vi "ShutterControl.vi"() -> ()   [LabVIEW 2019]
uses:
  <vilib>/DAQmx/write.llb/DAQmx Write (Analog DBL 1Chan 1Samp).vi
  <vilib>/DAQmx/miscellaneous.llb/DAQmx Fill In Error Info.vi
  <vilib>/DAQmx/create/channels.llb/DAQmx Create Channel (AO-Voltage-Basic).vi
  <vilib>/Analysis/1siggen.llb/Ramp Pattern by Delta.vi
  Driver/Newport ESP301/Newport ESP301.lvlib
  <vilib>/Analysis/NI_AALBase.lvlib
panel:
  in  "Dwell_positions":string[][](table)=[["-500", "3000"], ["-100", "3000"], ["0", "5000"], ["100", "5000"], ["500", "5000"], ["750", "10000"], ["1000", "10000"], ["", ""]]
  in  "Enable2":bool caption="Enable?"
  in  "Wait time [ms]":u32=1000 caption="Values <50 \nwon't work"
  out "StepSize [mm]":dbl=0.14989622900000002
  in  "stop 2":bool
  in  "StepSize [fs]":i32=1000
  in  "Enable?":bool
  out "a":waveform(dbl)(graph)={"t0"=timestamp(3675940489.011235 s since 1904-01-01), "dt"=1.0, "Y"=[-33.8895]}
  out "Waveform Chart":dbl(graph)=5.25341140860948
  out "x*y":dbl=-876.4751437142558
  in  "physical channels":tag="Dev1/ao1"
  out "DAC error":errorcluster
  out "ESP error":errorcluster
  out "run?":bool
  in  "set_vel":bool
  in  "velocity [fs/s]":dbl=333.564095198152
  in  "vel_mm":dbl=0.005 caption="velocity [mm/s]"
  out "meas. velocity":dbl
  in  "stop":bool
  out "output voltage":dbl
  in  "start":bool
  in  "go2p1":bool
  out "position [mm]":dbl=-33.8895
  in  "p2 [mm]":dbl=-0.707153771
  in  "p1 [mm]":dbl=-1.006946229
  in  "interpolate output":bool
  in  "Delta2 [fs]":dbl=999.9999999999999
  in  "Delta1 [fs]":dbl=-999.9999999999999
  in  "Reference [mm]":dbl=-0.85705
  in  "Axis (1)":i32=3 min=1 max=3
  in  "Serial Link (RS232)":enum16{"RS232", "USB"}(ring)
  in  "VISA resource name":refnum<visa-resource-name>="COM8"
  in  "main_close":bool
  # "Interface panel"
  # "Velocity panel"
  # "Positions panel"
  # "Equally spaced steps panel"
  # "Controls panel"
  # "User-defined steps panel"
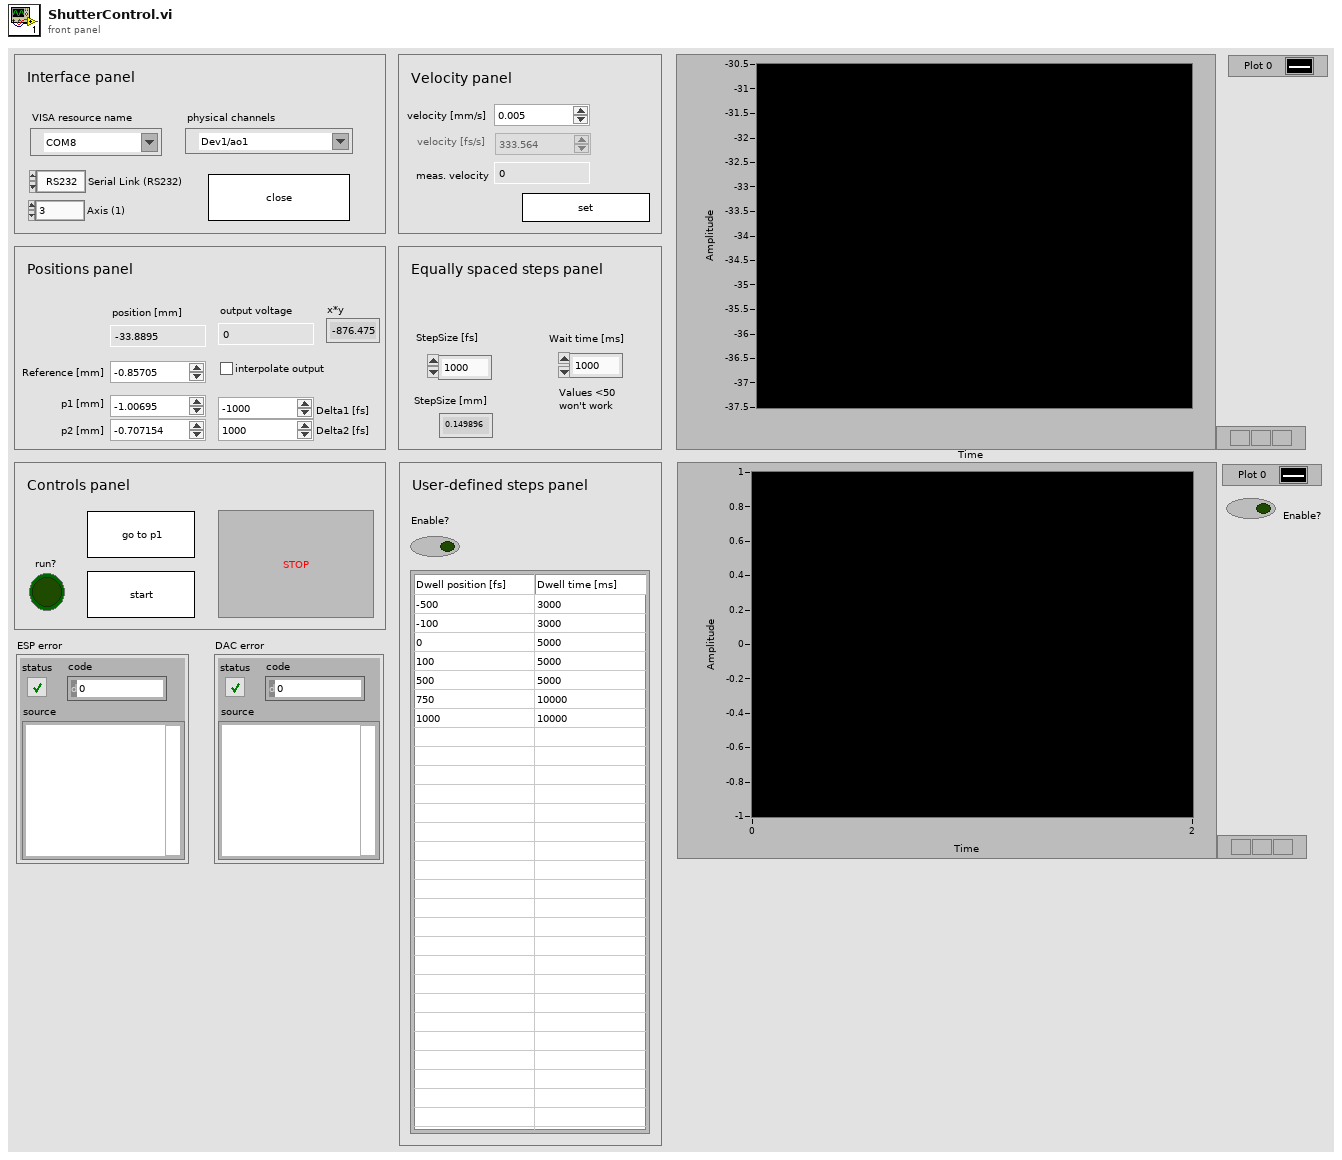
[diagram p1: front panel]
types:
  T1 = cluster{"dev1_data":refnum<queue>, "dev2_data":refnum<queue>}
  T2 = cluster{"dev1_cmd":refnum<queue>, "dev2_cmd":refnum<queue>}
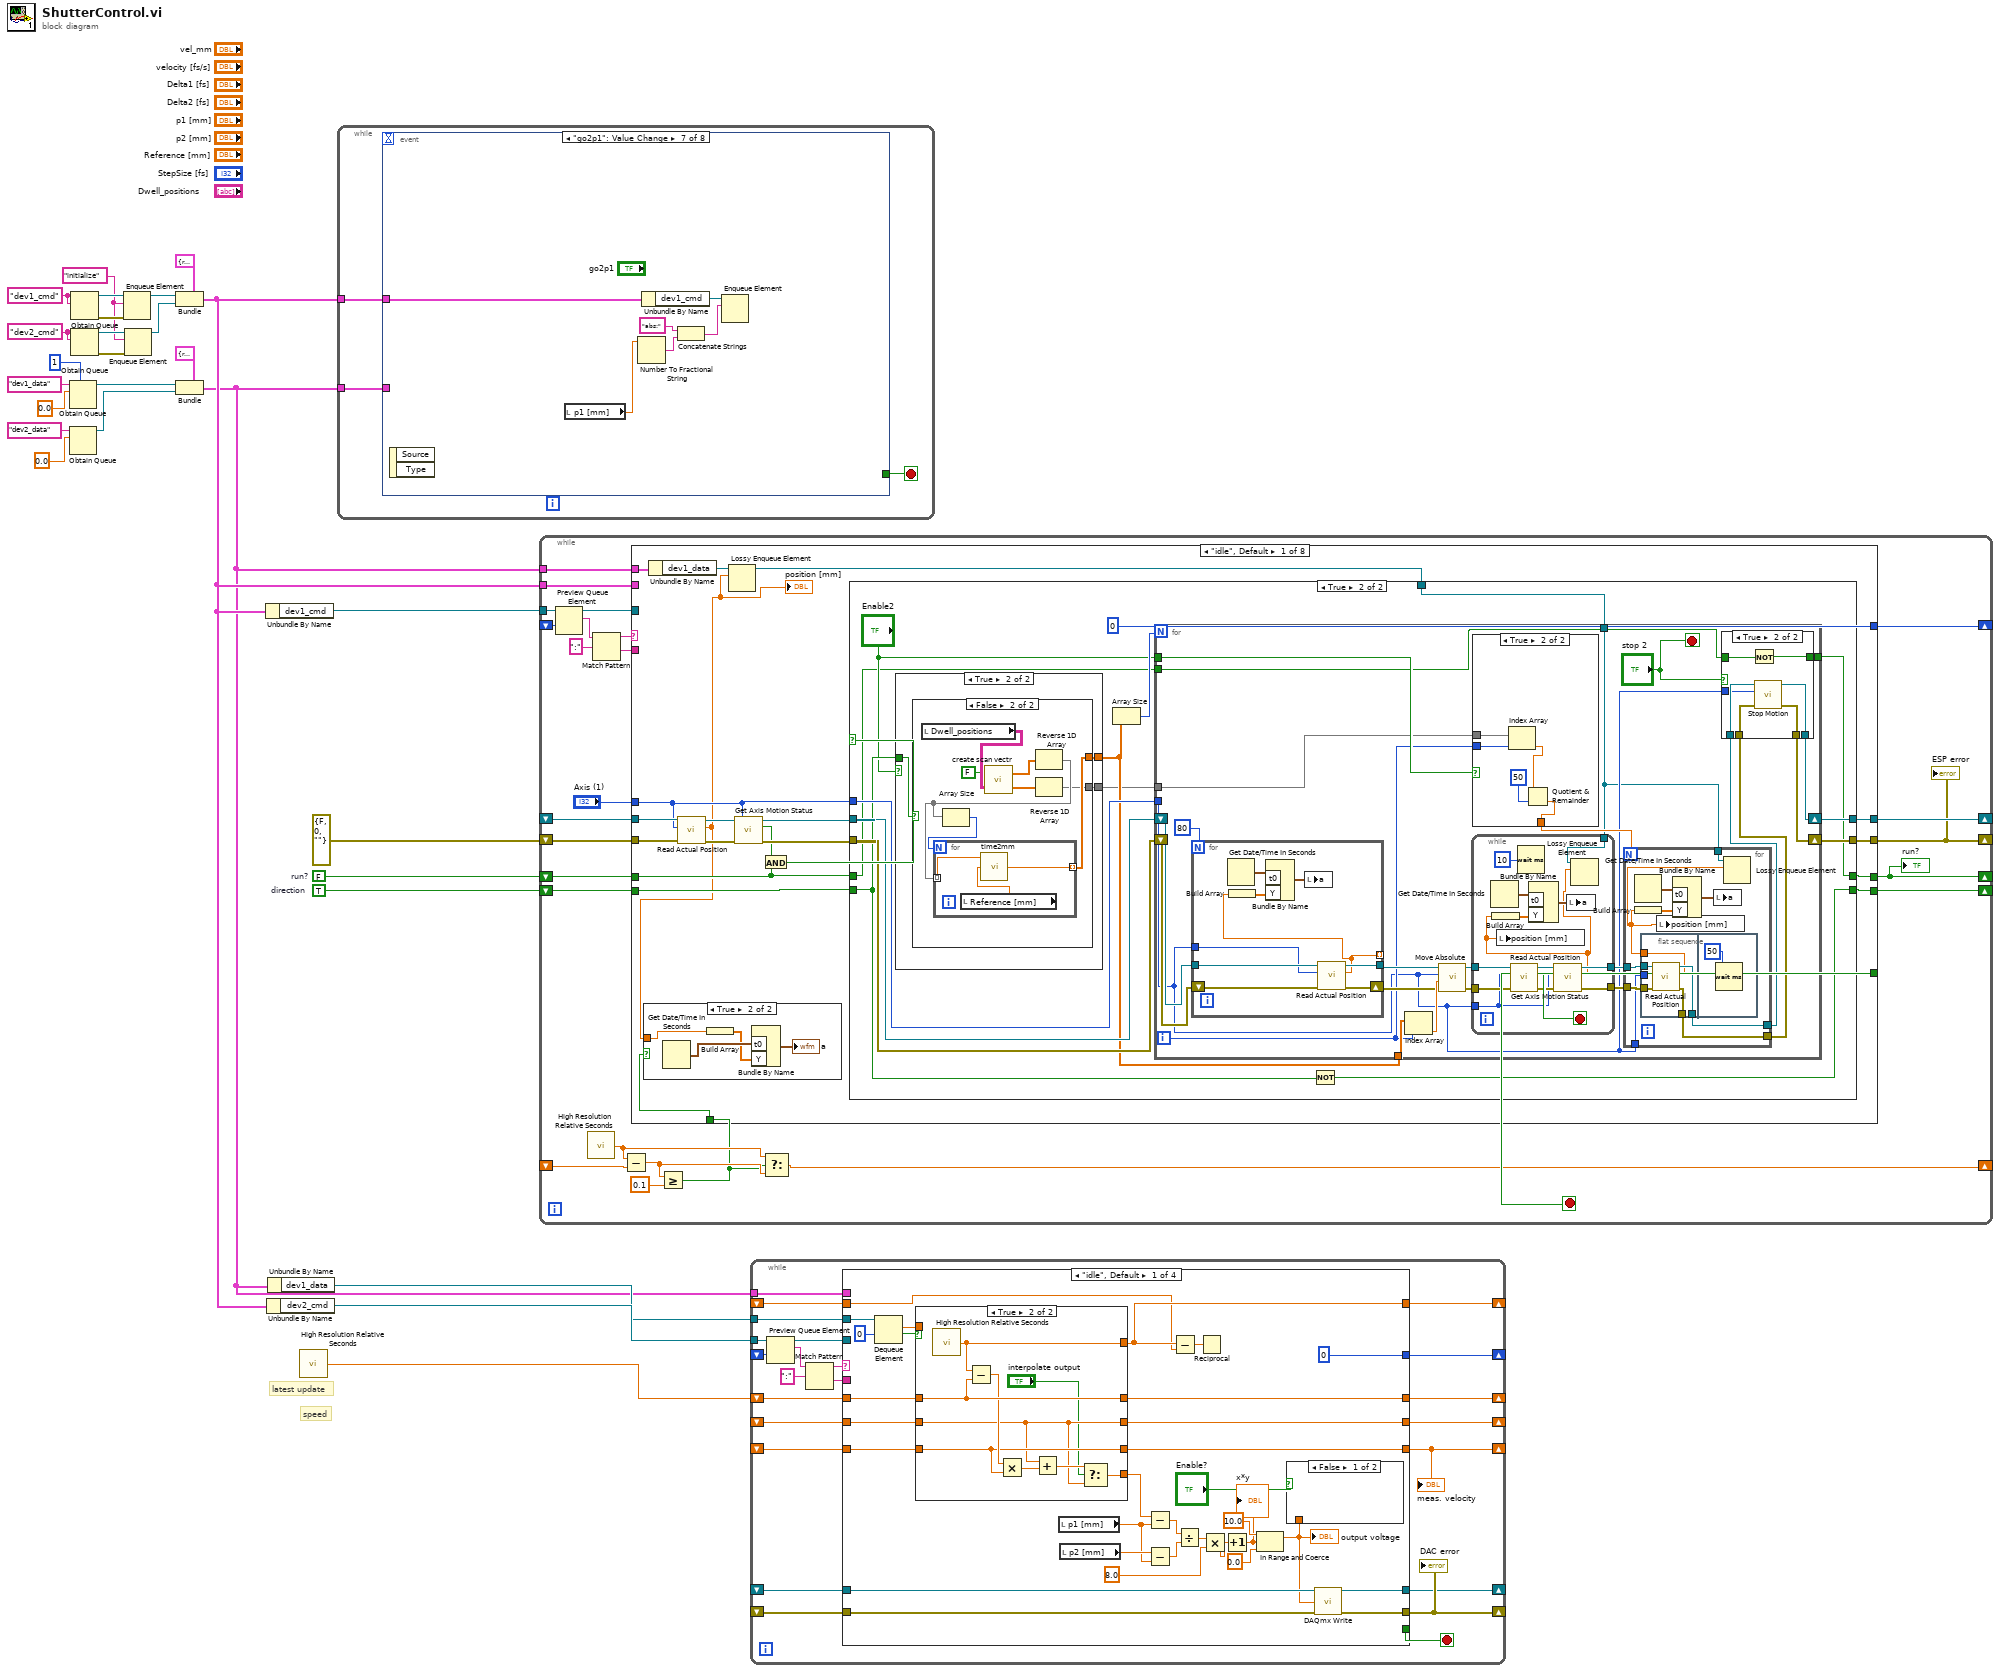
[diagram p0: block diagram]
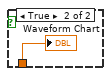
[diagram p2: hidden frame]
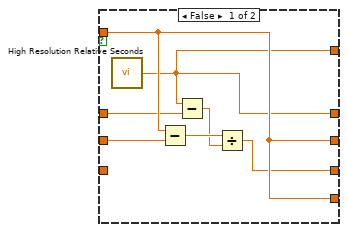
[diagram p3: hidden frame]
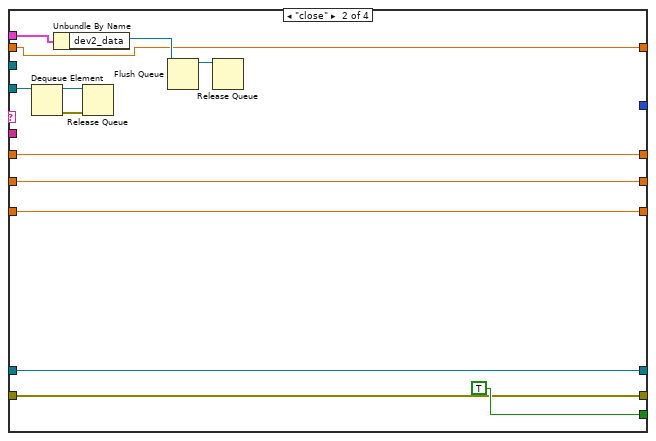
[diagram p4: hidden frame]
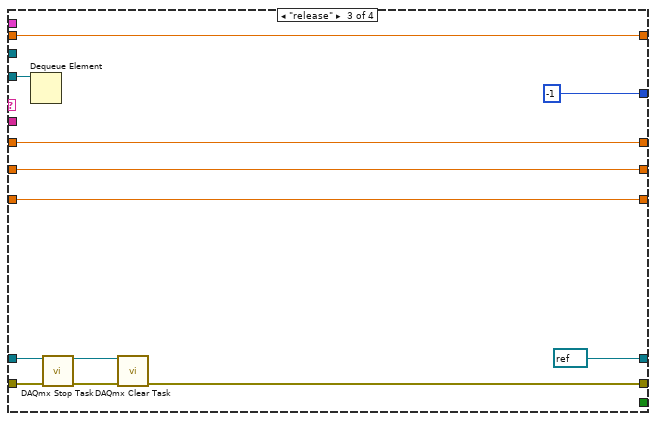
[diagram p5: hidden frame]
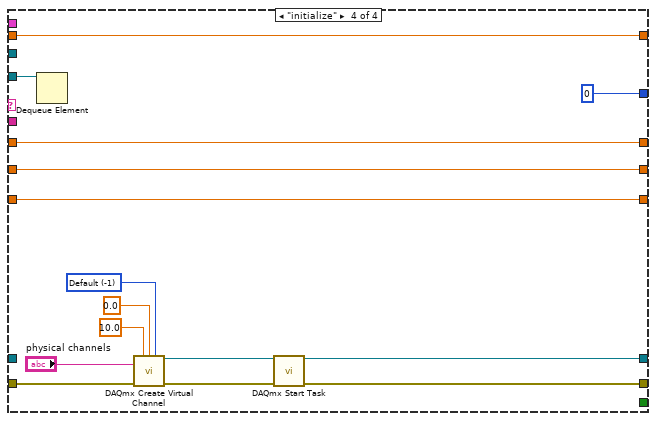
[diagram p6: hidden frame]
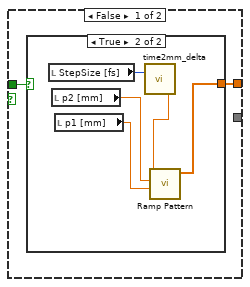
[diagram p9: hidden frame]
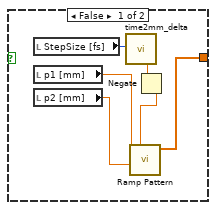
[diagram p10: hidden frame]
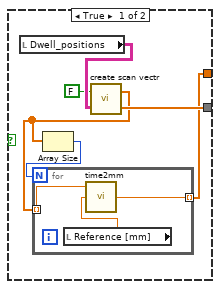
[diagram p11: hidden frame]
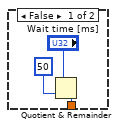
[diagram p13: hidden frame]
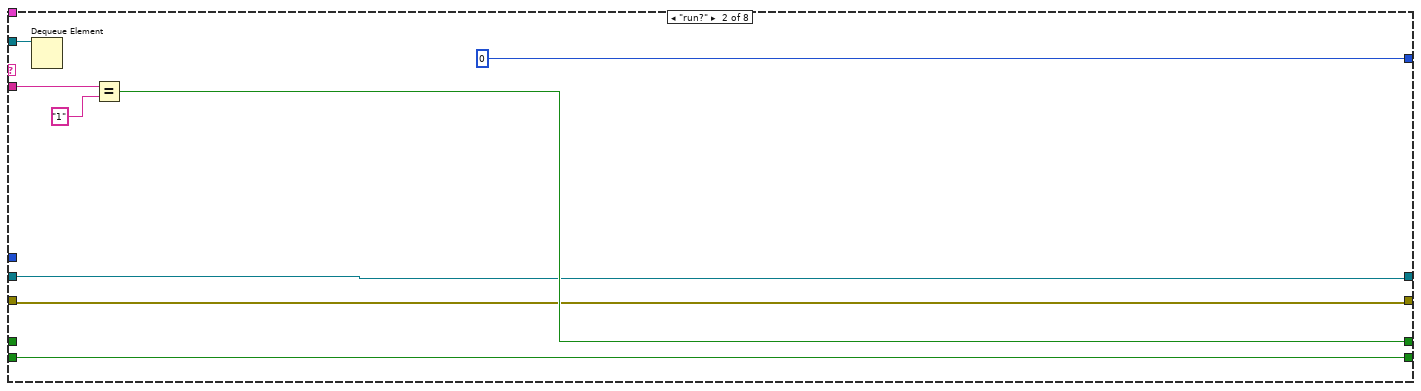
[diagram p14: hidden frame]
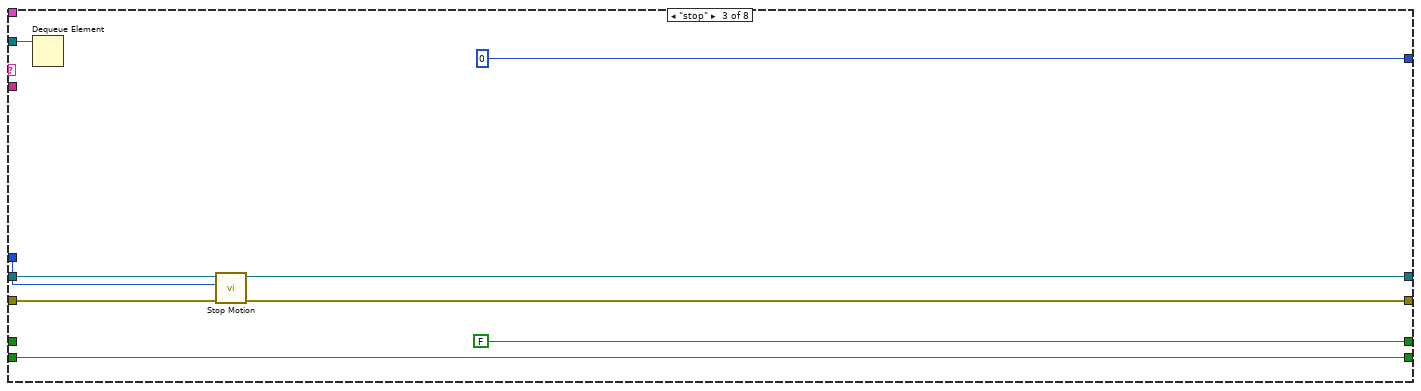
[diagram p15: hidden frame]
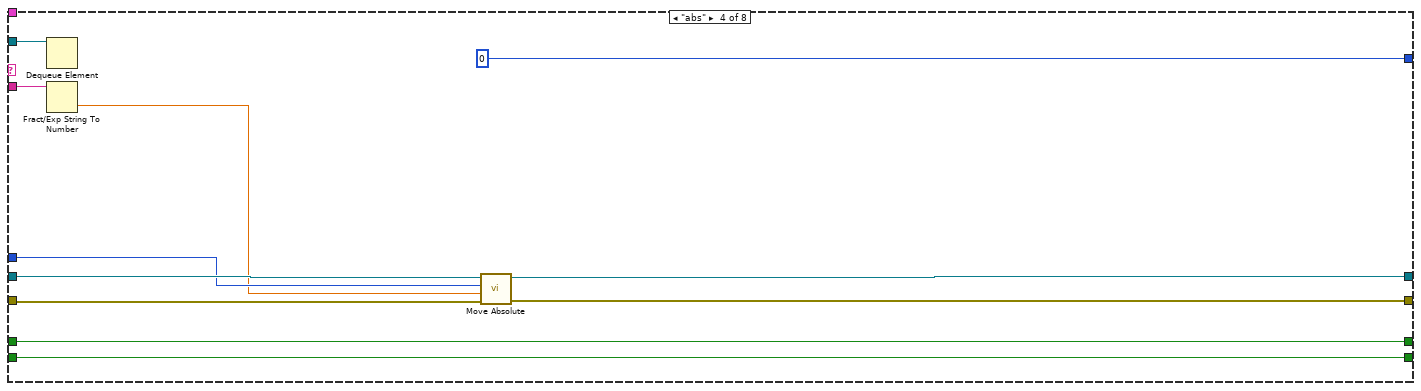
[diagram p16: hidden frame]
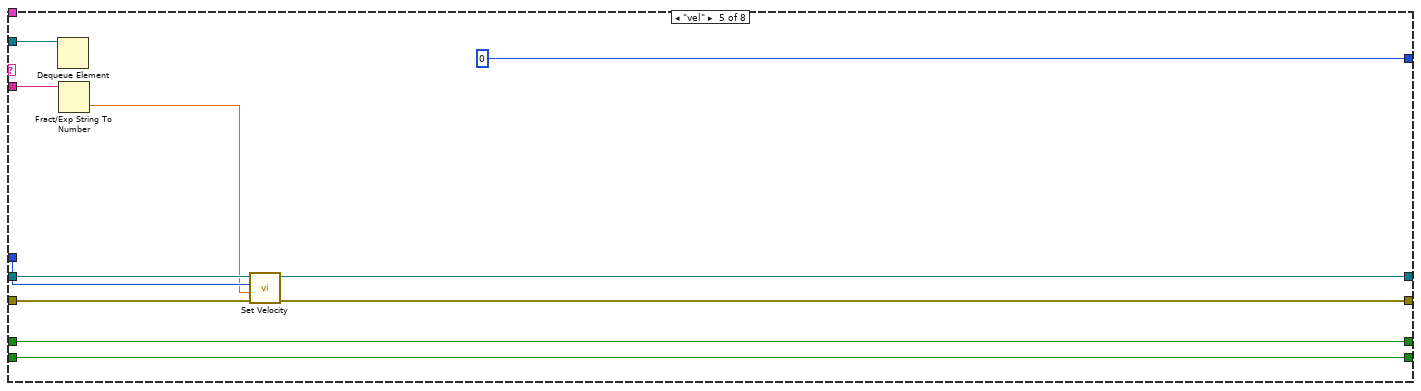
[diagram p17: hidden frame]
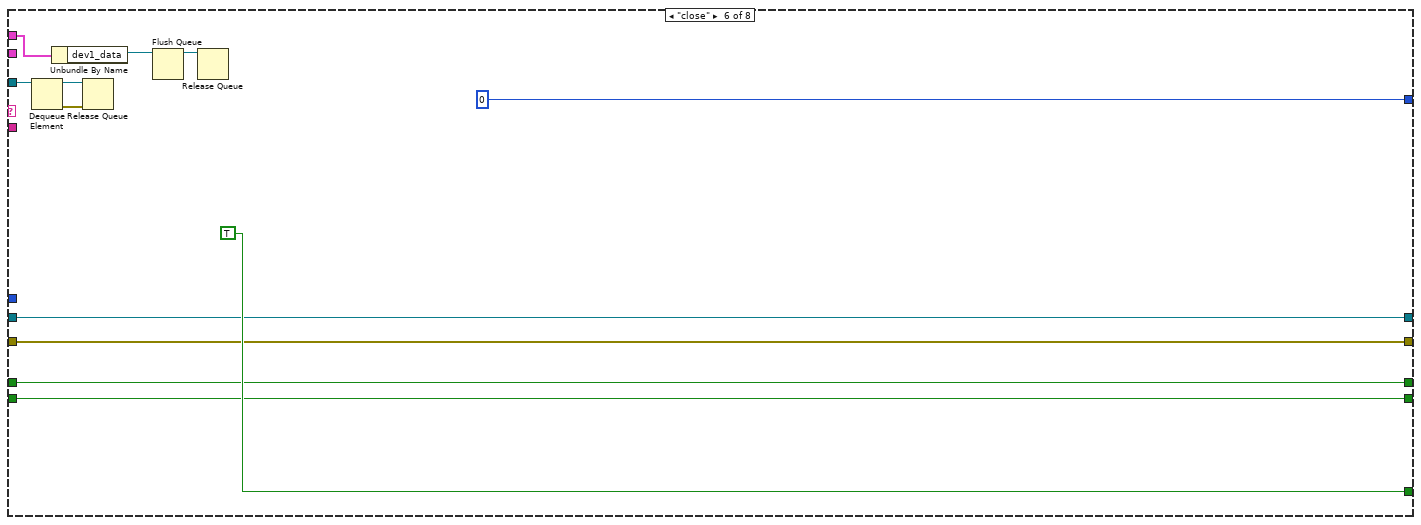
[diagram p18: hidden frame]
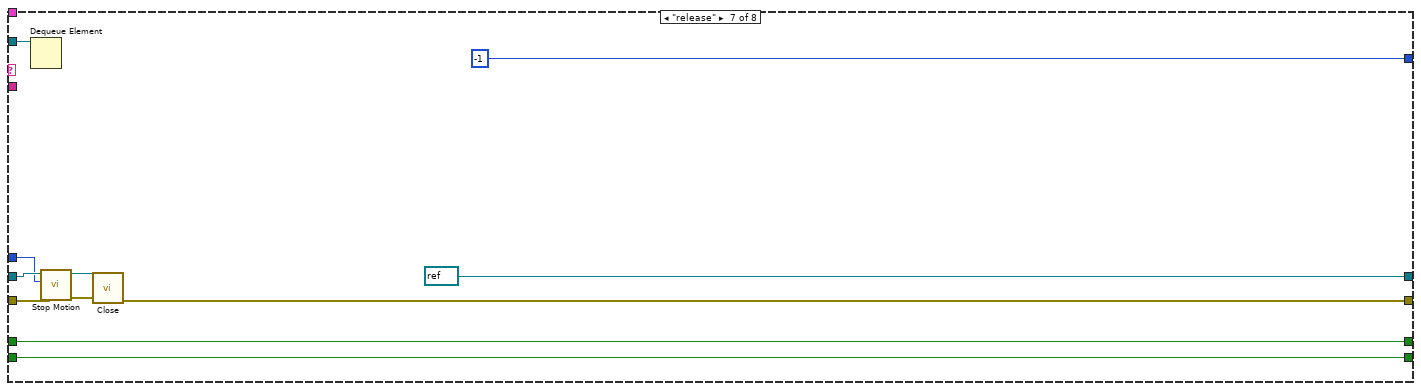
[diagram p19: hidden frame]
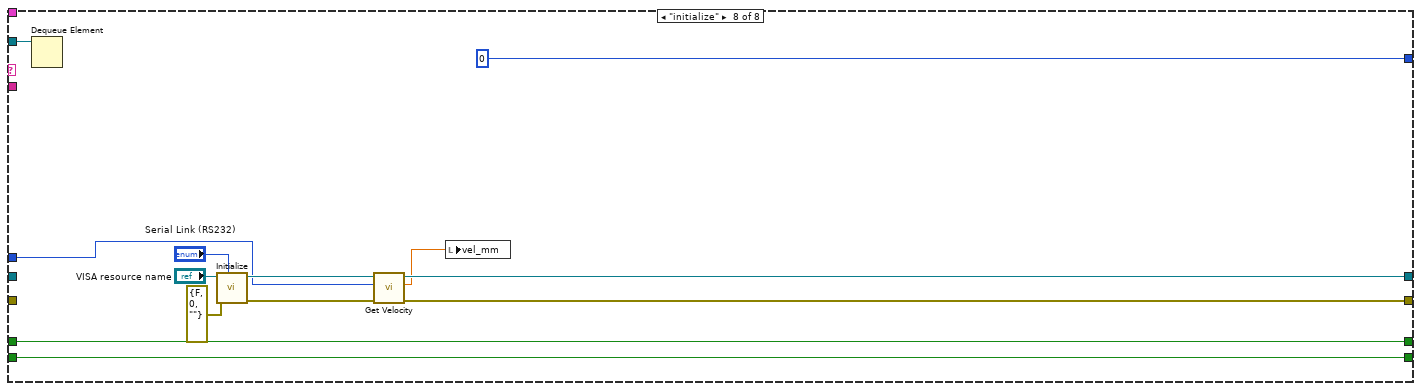
[diagram p20: hidden frame]
diagram:
  w1 = TRUE  # direction
  w4 = FALSE  # run?
  w15 = "dev2_cmd" ("name (unnamed)")
  w21 = "initialize" ("element")
  w16 = "dev1_cmd" ("name (unnamed)")
  # "speed"
  # "latest update"
  n1 = Obtain Queue(max queue size (-1, unlimited)=1, name (unnamed)="dev1_data", element data type=0.0) -> (queue out=w12:refnum<queue>)  [unwired: 2 in, 2 out]
  n2 = Obtain Queue(name (unnamed)="dev2_data", element data type=0.0) -> (queue out=w11:refnum<queue>)  [unwired: 3 in, 2 out]
  n3 = Obtain Queue(name (unnamed)=w16, element data type=w16) -> (queue out=w27:refnum<queue>, error out=w26:errorcluster)  [unwired: 3 in, 1 out]
  n4 = Obtain Queue(name (unnamed)=w15, element data type=w15) -> (queue out=w22:refnum<queue>, error out=w23:errorcluster)  [unwired: 3 in, 1 out]
  n5 = Enqueue Element(queue=w27, element=w21, error in (no error)=w26) -> (queue out=w24:refnum<queue>)  [unwired: 1 in, 2 out]
  n6 = Enqueue Element(queue=w22, element=w21, error in (no error)=w23) -> (queue out=w20:refnum<queue>)  [unwired: 1 in, 2 out]
  n7 = Bundle(cluster=T2 {"dev1_cmd"=refnum, "dev2_cmd"=refnum}, "dev1_cmd"=w24, "dev2_cmd"=w20) -> (w8:T2)
  n8 = Bundle(cluster=T1 {"dev1_data"=refnum, "dev2_data"=refnum}, "dev1_data"=w12, "dev2_data"=w11) -> (w2:T1)
  n9 = Unbundle By Name(w8) -> ("dev1_cmd"=w17:refnum<queue>)
  n10 = Unbundle By Name(w8) -> ("dev2_cmd"=w7:refnum<queue>)
  n11 = Unbundle By Name(w2) -> ("dev1_data"=w6:refnum<queue>)
  n12 = call <vilib>:"High Resolution Relative Seconds.vi"() -> ("relative seconds"=w5:dbl)
  n13 = while {
    tunnel: w8 -> [w30]
    tunnel: w2 -> [w29]
    stop <- w28 stop-if-true
    n14 = event shown="[6] \"go2p1\": Value Change" {
      selector: _ -> [_ _ _ _ _ _ _ _]
      dyn-events: _ -> [_ _ _ _ _ _ _ _]
      timeout: _ -> [_ _ _ _ _ _ _ _]
      tunnel: w30 -> [_ w34 _ _ w46 _ w64 w67]
      tunnel: w29 -> [_ _ _ _ _ _ _ _]
      tunnel: [_ _ _ _ _ _ _ TRUE] -> w28
      event Timeout {
        n15 = event-data() -> ()  [unwired: 1 in, 1 out]
      }
      event "start", "stop": Value Change {
        n16 = event-data() -> ()  [unwired: 1 in, 1 out]
        n17 = Boolean To (0,1)(Boolean="start") -> (0, 1=w32:i16)
        n18 = Number To Decimal String(number=w32) -> (decimal integer string=w31:string)  [unwired: 1 in]
        n19 = Unbundle By Name(w34) -> ("dev1_cmd"=w37:refnum<queue>)
        n20 = Concatenate Strings("run?:" ("string"), w31) -> (w36:string)
        n21 = Enqueue Element(queue=w37, element=w36) -> ()  [unwired: 2 in, 3 out]
      }
      event "StepSize [fs]": Value Change {
        n22 = event-data() -> ("NewVal"=w38:i32)  [unwired: 1 in, 5 out]
        n23 = call "time2mm_delta.vi"("Delta time"=w38) -> ("Delta position (mm)"=→"StepSize [mm]":dbl)  [unwired: 2 in]
      }
      event "Delta1 [fs]", "Delta2 [fs]": Value Change {
        n24 = event-data() -> ()  [unwired: 1 in, 1 out]
        n25 = local read "Reference [mm]"() -> (w41:dbl)
        n26 = local read "Delta2 [fs]"() -> (w42:dbl)
        n27 = local read "Delta1 [fs]"() -> (w44:dbl)
        n28 = call "time2mm.vi"("Offset (mm)"=w41, "time"=w44) -> ("position (mm)"=w43:dbl)  [unwired: 1 in]
        n29 = call "time2mm.vi"("Offset (mm)"=w41, "time"=w42) -> ("position (mm)"=w40:dbl)  [unwired: 1 in]
        n30 = local write "p2 [mm]"(w40) -> ()
        n31 = local write "p1 [mm]"(w43) -> ()
      }
      event "set_vel": Value Change {
        n32 = event-data() -> ()  [unwired: 1 in, 2 out]
        n33 = local read "vel_mm"() -> (w45:dbl)
        n34 = Number To Fractional String(number=w45) -> (F-format string=w49:string)  [unwired: 3 in]
        n35 = Unbundle By Name(w46) -> ("dev1_cmd"=w50:refnum<queue>)
        n36 = Concatenate Strings("vel:" ("string"), w49) -> (w48:string)
        n37 = Enqueue Element(queue=w50, element=w48) -> ()  [unwired: 2 in, 3 out]
      }
      event "p1 [mm]", "p2 [mm]", "Reference [mm]", "vel_mm": Value Change {
        n38 = event-data() -> ()  [unwired: 1 in, 2 out]
        n39 = local read "Reference [mm]"() -> (w56:dbl)
        n40 = local read "vel_mm"() -> (w53:dbl)
        n41 = local read "p1 [mm]"() -> (w57:dbl)
        n42 = local read "p2 [mm]"() -> (w58:dbl)
        n43 = call "mm2time.vi"("Offset (mm)"=0.0, "distance (mm)"=w53) -> ("time in fs"=w52:dbl)  [unwired: 1 in]
        n44 = call "mm2time.vi"("Offset (mm)"=w56, "distance (mm)"=w57) -> ("time in fs"=w54:dbl)  [unwired: 1 in]
        n45 = call "mm2time.vi"("Offset (mm)"=w56, "distance (mm)"=w58) -> ("time in fs"=w55:dbl)  [unwired: 1 in]
        n46 = local write "velocity [fs/s]"(w52) -> ()
        n47 = local write "Delta1 [fs]"(w54) -> ()
        n48 = local write "Delta2 [fs]"(w55) -> ()
      }
      event "go2p1": Value Change {
        n49 = event-data() -> ()  [unwired: 1 in, 2 out]
        n50 = local read "p1 [mm]"() -> (w59:dbl)
        n51 = Number To Fractional String(number=w59) -> (F-format string=w62:string)  [unwired: 3 in]
        n52 = Unbundle By Name(w64) -> ("dev1_cmd"=w63:refnum<queue>)
        n53 = Concatenate Strings("abs:" ("string"), w62) -> (w60:string)
        n54 = Enqueue Element(queue=w63, element=w60) -> ()  [unwired: 2 in, 3 out]
      }
      event "main_close": Value Change {
        n55 = event-data() -> ()  [unwired: 1 in, 1 out]
        n56 = Cluster To Array(cluster=w67) -> (array=w66:refnum<queue>[])
        n57 = for {
          tunnel: w66 -> [w72] mode=indexing
          n58 = Flush Queue(queue=w72) -> (queue out=w68:refnum<queue>)  [unwired: 1 in, 2 out]
          n59 = Enqueue Element(queue=w68, element="release") -> (queue out=w70:refnum<queue>)  [unwired: 2 in, 2 out]
          n60 = Enqueue Element(queue=w70, element="close") -> ()  [unwired: 2 in, 3 out]
        }
      }
    }
  }
  n61 = while {
    tunnel: w8 -> [w93]
    tunnel: w17 -> [w98]
    tunnel: w2 -> [w90]
    shift-right: [w88] -> _
    shift-left: _ -> [w89]
    shift-right: [w87] -> _
    shift-left: _ -> [w84]
    shift-right: [w86] -> _
    shift-left: errorcluster {"status"=FALSE, "code"=0, "source"=""} ("error out") -> [w85]
    shift-right: [w81] -> _
    shift-left: w4 -> [w82]
    shift-right: [w79] -> _
    shift-left: w1 -> [w80]
    shift-right: [w73] -> _
    shift-left: _ -> [w78]
    stop <- w91 stop-if-true
    n62 = Preview Queue Element(queue=w98, timeout in ms (-1)=w89) -> (queue out=w92:refnum<queue>, element=w97:string)  [unwired: 1 in, 2 out]
    n63 = call <vilib>:"High Resolution Relative Seconds.vi"() -> ("relative seconds"=w75:dbl)
    n64 = Match Pattern(string=w97, regular expression=":") -> (before substring=w95:string, after substring=w94:string)  [unwired: 1 in, 2 out]
    n65 = Subtract(x=w75, y=w78) -> (x-y=w76:dbl)
    n66 = Greater Or Equal?(x=w76, y=0.1) -> (x >= y?=w74:bool)
    n67 = case shown="\"idle\", Default" w95 {
      tunnel: w94 -> [_ w267 _ w286 w293 _ _ _]
      tunnel: w93 -> [_ _ _ _ _ _ _ _]
      tunnel: w92 -> [_ w265 w269 w287 w291 w310 w320 w330]
      tunnel: [_ _ _ _ _ TRUE _ _] -> w91
      tunnel: w90 -> [w118 _ _ _ _ w302 _ _]
      tunnel: [0 0 0 0 0 0 -1 0] -> w88
      tunnel: [w116 w260 w274 w283 w298 w306 refnum<visa-resource-name> refnum ("VISA resource name out") w326] -> w87
      tunnel: [w115 w261 w273 w282 w297 w305 w319 w325] -> w86
      tunnel: w85 -> [w113 w261 w275 w284 w296 w305 w315 _]
      tunnel: w84 -> [w114 w260 w276 w285 w295 w306 w312 _]
      tunnel: "Axis (1)" -> [w104 _ w272 w281 w294 _ w311 w327]
      tunnel: w82 -> [w102 _ _ w278 w289 w303 w317 w331]
      tunnel: [w110 w263 FALSE ("run?") w278 w289 w303 w317 w331] -> w81
      tunnel: w80 -> [w111 w262 w268 w277 w288 w299 w316 w322]
      tunnel: [w112 w262 w268 w277 w288 w299 w316 w322] -> w79
      tunnel: w74 -> [w99 _ _ _ _ _ _ _]
      frame "idle", Default {
        n68 = Unbundle By Name(w118) -> ("dev1_data"=w117:refnum<queue>)
        n69 = call "Read Actual Position.vi"("error in (no error)"=w113, "Axis (1)"=w104, "VISA resource name"=w114) -> ("error out"=w107:errorcluster, "Position (units)"=w100:dbl, "VISA resource name out"=w108:refnum<visa-resource-name>)  [unwired: 2 in]
        "position [mm]" <- w100
        n70 = case shown="True" w99 {
          tunnel: w100 -> [_ w123]
          frame False {
          }
          frame True {
            n71 = Get Date/Time In Seconds() -> (seconds since 1Jan1904=w122:timestamp)
            n72 = Build Array(w123) -> (w121:dbl[])
            n73 = Bundle By Name("t0"=w122, "Y"=w121) -> (→"a":waveform(dbl))  [unwired: 1 in]
          }
        }
        n74 = Lossy Enqueue Element(queue=w117, element=w100) -> (queue out=w109:refnum<queue>)  [unwired: 1 in, 3 out]
        n75 = call "Get Axis Motion Status.vi"("error in (no error)"=w107, "Axis (1)"=w104, "VISA resource name"=w108) -> ("error out"=w105:errorcluster, "Motion Done"=w103:bool, "VISA resource name out"=w106:refnum<visa-resource-name>)  [unwired: 2 in]
        n76 = And(x=w103, y=w102) -> (x .and. y?=w101:bool)
        n77 = case shown="True" w101 {
          tunnel: w106 -> [w127 w140]
          tunnel: w105 -> [w126 w141]
          tunnel: [w127 w139] -> w116
          tunnel: [w126 w138] -> w115
          tunnel: w104 -> [_ w137]
          tunnel: [w125 w136] -> w112
          tunnel: w111 -> [w125 w135]
          tunnel: w102 -> [w124 w130]
          tunnel: [w124 w129] -> w110
          tunnel: w109 -> [_ w128]
          frame False {
          }
          frame True {
            n78 = case shown="True" "Enable2" {
              tunnel: w135 -> [w143 w155]
              tunnel: [w142 w156] -> w134
              tunnel: [_ w157] -> w131
              frame False {
                n79 = case shown="True" w143 {
                  tunnel: [w147 w152] -> w142
                  frame False {
                    n80 = local read "StepSize [fs]"() -> (w144:i32)
                    n81 = local read "p1 [mm]"() -> (w149:dbl)
                    n82 = local read "p2 [mm]"() -> (w148:dbl)
                    n83 = call "time2mm_delta.vi"("Delta time"=w144) -> ("Delta position (mm)"=w145:dbl)  [unwired: 2 in]
                    n84 = Negate(x=w145) -> (-x=w146:dbl)
                    n85 = call-poly <vilib>:"Ramp Pattern.vi"("start"=w148, "end"=w149, "delta"=w146) -> ("Ramp Pattern"=w147:dbl[])  [unwired: 6 in, 2 out]
                  }
                  frame True {
                    n86 = local read "StepSize [fs]"() -> (w150:i32)
                    n87 = local read "p2 [mm]"() -> (w153:dbl)
                    n88 = local read "p1 [mm]"() -> (w154:dbl)
                    n89 = call "time2mm_delta.vi"("Delta time"=w150) -> ("Delta position (mm)"=w151:dbl)  [unwired: 2 in]
                    n90 = call-poly <vilib>:"Ramp Pattern.vi"("start"=w154, "end"=w153, "delta"=w151) -> ("Ramp Pattern"=w152:dbl[])  [unwired: 6 in, 2 out]
                  }
                }
              }
              frame True {
                n91 = case shown="False" w155 {
                  tunnel: [w161 w167] -> w157
                  tunnel: [w160 w172] -> w156
                  frame True {
                    n92 = local read "Dwell_positions"() -> (w163:string[][])
                    n93 = call "create scan vectr.vi"("Table Control"=w163, "waypoint mode?"=FALSE) -> ("Array 2"=w161:dbl[], "Array"=w159:dbl[])
                    n94 = Array Size(array=w159) -> (size(s)=w158:i32)
                    n95 = for {
                      N: w158 -> [_]
                      tunnel: w159 -> [w166] mode=indexing
                      tunnel: [w165] -> w160 mode=indexing
                      n96 = local read "Reference [mm]"() -> (w164:dbl)
                      n97 = call "time2mm.vi"("Offset (mm)"=w164, "time"=w166) -> ("position (mm)"=w165:dbl)  [unwired: 1 in]
                    }
                  }
                  frame False {
                    n98 = local read "Dwell_positions"() -> (w174:string[][])
                    n99 = call "create scan vectr.vi"("Table Control"=w174, "waypoint mode?"=FALSE) -> ("Array 2"=w168:dbl[], "Array"=w169:dbl[])
                    n100 = Reverse 1D Array(array=w169) -> (reversed array=w170:dbl[])
                    n101 = Array Size(array=w170) -> (size(s)=w171:i32)
                    n102 = for {
                      N: w171 -> [_]
                      tunnel: w170 -> [w177] mode=indexing
                      tunnel: [w176] -> w172 mode=indexing
                      n103 = local read "Reference [mm]"() -> (w175:dbl)
                      n104 = call "time2mm.vi"("Offset (mm)"=w175, "time"=w177) -> ("position (mm)"=w176:dbl)  [unwired: 1 in]
                    }
                    n105 = Reverse 1D Array(array=w168) -> (reversed array=w167:dbl[])
                  }
                }
              }
            }
            n106 = Array Size(array=w134) -> (size(s)=w133:i32)
            n107 = for {
              N: w133 -> [_]
              tunnel: w137 -> [w181]
              tunnel: w134 -> [w196]
              shift-right: [w183] -> w138
              shift-left: w141 -> [w200]
              shift-right: [w185] -> w139
              shift-left: w140 -> [w199]
              tunnel: "Enable2" -> [w189]
              tunnel: w131 -> [w187]
              tunnel: w130 -> [w180]
              tunnel: [w179] -> w129
              tunnel: w128 -> [w178]
              i -> [w188]
              stop <- "stop 2" stop-if-true
              n108 = for {
                N: 80 -> [_]
                tunnel: w199 -> [w259]
                tunnel: [w258] -> w198
                shift-right: [w255] -> w193
                shift-left: w200 -> [w257]
                tunnel: w181 -> [w256]
                tunnel: [w252] -> _ mode=indexing
                n109 = Get Date/Time In Seconds() -> (seconds since 1Jan1904=w253:timestamp)
                n110 = call "Read Actual Position.vi"("error in (no error)"=w257, "Axis (1)"=w256, "VISA resource name"=w259) -> ("error out"=w255:errorcluster, "Position (units)"=w252:dbl, "VISA resource name out"=w258:refnum<visa-resource-name>)  [unwired: 2 in]
                n111 = Build Array(w252) -> (w254:dbl[])
                n112 = Bundle By Name("t0"=w253, "Y"=w254) -> (w251:waveform(dbl))  [unwired: 1 in]
                n113 = local write "a"(w251) -> ()
              }
              n114 = Index Array(array=w196, index=w188) -> (element=w197:dbl)
              n115 = call "Move Absolute.vi"("error in (no error)"=w193, "Position (0 units)"=w197, "Axis (1)"=w181, "VISA resource name"=w198) -> ("error out"=w194:errorcluster, "VISA resource name out"=w195:refnum<visa-resource-name>)  [unwired: 2 in]
              n116 = while {
                tunnel: w195 -> [w250]
                tunnel: [w245] -> w190
                tunnel: w194 -> [w249]
                tunnel: [w243] -> w191
                tunnel: w181 -> [w242]
                tunnel: w178 -> [w237]
                stop <- w247 stop-if-true
                n117 = Get Date/Time In Seconds() -> (seconds since 1Jan1904=w241:timestamp)
                n118 = call "Get Axis Motion Status.vi"("error in (no error)"=w249, "Axis (1)"=w242, "VISA resource name"=w250) -> ("error out"=w244:errorcluster, "Motion Done"=w247:bool, "VISA resource name out"=w246:refnum<visa-resource-name>)  [unwired: 2 in]
                n119 = Wait (ms)(milliseconds to wait=10) -> ()  [unwired: 1 out]
                n120 = call "Read Actual Position.vi"("error in (no error)"=w244, "Axis (1)"=w242, "VISA resource name"=w246) -> ("error out"=w243:errorcluster, "Position (units)"=w238:dbl, "VISA resource name out"=w245:refnum<visa-resource-name>)  [unwired: 2 in]
                n121 = Build Array(w238) -> (w240:dbl[])
                n122 = local write "position [mm]"(w238) -> ()
                n123 = Bundle By Name("t0"=w241, "Y"=w240) -> (w239:waveform(dbl))  [unwired: 1 in]
                n124 = local write "a"(w239) -> ()
                n125 = Lossy Enqueue Element(queue=w237, element=w238) -> ()  [unwired: 1 in, 4 out]
              }
              n126 = case shown="True" w189 {
                tunnel: [w212 w218] -> w192
                tunnel: w188 -> [_ w216]
                tunnel: w187 -> [_ w215]
                frame False {
                  n127 = Quotient & Remainder(x="Wait time [ms]", y=50) -> (floor(x/y)=w212:u32)  [unwired: 1 out]
                }
                frame True {
                  n128 = Index Array(array=w215, index=w216) -> (element=w217:dbl)
                  n129 = Quotient & Remainder(x=w217, y=50) -> (floor(x/y)=w218:dbl)  [unwired: 1 out]
                }
              }
              n130 = for {
                N: w192 -> [_]
                tunnel: w191 -> [w229]
                tunnel: [w228] -> w184
                tunnel: w190 -> [w227]
                tunnel: [w226] -> w186
                tunnel: w181 -> [w225]
                tunnel: w178 -> [w220]
                n131 = Get Date/Time In Seconds() -> (seconds since 1Jan1904=w223:timestamp)
                n132 = Build Array(w221) -> (w224:dbl[])
                n133 = flat-sequence {
                  tunnel: w229 -> [w235]
                  tunnel: [w234] -> w228
                  tunnel: w227 -> [w233]
                  tunnel: [w232] -> w226
                  tunnel: w225 -> [w231]
                  tunnel: [w230] -> w221
                  frame #0 {
                    n134 = call "Read Actual Position.vi"("error in (no error)"=w235, "Axis (1)"=w231, "VISA resource name"=w233) -> ("error out"=w234:errorcluster, "Position (units)"=w230:dbl, "VISA resource name out"=w232:refnum<visa-resource-name>)  [unwired: 2 in]
                  }
                  frame #1 {
                    n135 = Wait (ms)(milliseconds to wait=50) -> ()  [unwired: 1 out]
                  }
                }
                n136 = local write "position [mm]"(w221) -> ()
                n137 = Bundle By Name("t0"=w223, "Y"=w224) -> (w222:waveform(dbl))  [unwired: 1 in]
                n138 = local write "a"(w222) -> ()
                n139 = Lossy Enqueue Element(queue=w220, element=w221) -> ()  [unwired: 1 in, 4 out]
              }
              n140 = case shown="True" "stop 2" {
                tunnel: w186 -> [w204 w211]
                tunnel: [w204 w210] -> w185
                tunnel: w184 -> [w203 w209]
                tunnel: [w203 w208] -> w183
                tunnel: w181 -> [_ w207]
                tunnel: w180 -> [w202 w206]
                tunnel: [w202 w205] -> w179
                frame False {
                }
                frame True {
                  n141 = Not(x=w206) -> (.not. x?=w205:bool)
                  n142 = call "Stop Motion.vi"("error in (no error)"=w209, "Axis (1)"=w207, "VISA resource name"=w211) -> ("error out"=w208:errorcluster, "VISA resource name out"=w210:refnum<visa-resource-name>)  [unwired: 3 in]
                }
              }
            }
            n143 = Not(x=w135) -> (.not. x?=w136:bool)
          }
        }
      }
      frame "run?" {
        n144 = Dequeue Element(queue=w265) -> ()  [unwired: 2 in, 4 out]
        n145 = Equal?(x=w267, y="1") -> (x = y?=w263:bool)
      }
      frame "stop" {
        n146 = Dequeue Element(queue=w269) -> ()  [unwired: 2 in, 4 out]
        n147 = call "Stop Motion.vi"("error in (no error)"=w275, "Axis (1)"=w272, "VISA resource name"=w276) -> ("error out"=w273:errorcluster, "VISA resource name out"=w274:refnum<visa-resource-name>)  [unwired: 3 in]
      }
      frame "abs" {
        n148 = Dequeue Element(queue=w287) -> ()  [unwired: 2 in, 4 out]
        n149 = Fract/Exp String To Number(string=w286) -> (number=w280:dbl)  [unwired: 3 in, 1 out]
        n150 = call "Move Absolute.vi"("error in (no error)"=w284, "Position (0 units)"=w280, "Axis (1)"=w281, "VISA resource name"=w285) -> ("error out"=w282:errorcluster, "VISA resource name out"=w283:refnum<visa-resource-name>)  [unwired: 2 in]
      }
      frame "vel" {
        n151 = Dequeue Element(queue=w291) -> ()  [unwired: 2 in, 4 out]
        n152 = Fract/Exp String To Number(string=w293) -> (number=w292:dbl)  [unwired: 3 in, 1 out]
        n153 = call "Set Velocity.vi"("error in (no error)"=w296, "Velocity (units/s)"=w292, "Axis (1)"=w294, "VISA resource name"=w295) -> ("error out"=w297:errorcluster, "VISA resource name out"=w298:refnum<visa-resource-name>)  [unwired: 2 in]
      }
      frame "close" {
        n154 = Dequeue Element(queue=w310) -> (queue out=w309:refnum<queue>, error out=w308:errorcluster)  [unwired: 2 in, 2 out]
        n155 = Unbundle By Name(w302) -> ("dev1_data"=w300:refnum<queue>)
        n156 = Release Queue(queue=w309, error in (no error)=w308) -> ()  [unwired: 1 in, 3 out]
        n157 = Flush Queue(queue=w300) -> (queue out=w301:refnum<queue>)  [unwired: 1 in, 2 out]
        n158 = Release Queue(queue=w301) -> ()  [unwired: 2 in, 3 out]
      }
      frame "release" {
        n159 = Dequeue Element(queue=w320) -> ()  [unwired: 2 in, 4 out]
        n160 = call "Stop Motion.vi"("error in (no error)"=w315, "Axis (1)"=w311, "VISA resource name"=w312) -> ("error out"=w314:errorcluster, "VISA resource name out"=w313:refnum<visa-resource-name>)  [unwired: 3 in]
        n161 = call "Close.vi"("error in (no error)"=w314, "VISA resource name"=w313) -> ("error out"=w319:errorcluster)  [unwired: 9 in]
      }
      frame "initialize" {
        n162 = Dequeue Element(queue=w330) -> ()  [unwired: 2 in, 4 out]
        n163 = call "Initialize.vi"("VISA resource name"="VISA resource name", "error in (no error)"=errorcluster {"status"=FALSE, "code"=0, "source"=""}, "Serial Link (RS232)"="Serial Link (RS232)") -> ("VISA resource name out"=w329:refnum<visa-resource-name>, "error out"=w328:errorcluster)  [unwired: 6 in]
        n164 = call "Get Velocity.vi"("error in (no error)"=w328, "Axis (1)"=w327, "VISA resource name"=w329) -> ("error out"=w325:errorcluster, "Velocity (units/s)"=w324:dbl, "VISA resource name out"=w326:refnum<visa-resource-name>)  [unwired: 2 in]
        n165 = local write "vel_mm"(w324) -> ()
      }
    }
    "run?" <- w81
    "ESP error" <- w86
    n166 = Select(t=w75, s=w74, f=w76) -> (s? t:f=w73:dbl)
  }
  n167 = while {
    shift-right: [w350] -> _
    shift-left: _ -> [w351]
    shift-right: [w349] -> _
    shift-left: _ -> [w348]
    tunnel: w7 -> [w347]
    shift-right: [w346] -> _
    shift-left: _ -> [w345]
    tunnel: w6 -> [w344]
    shift-right: [w343] -> _
    shift-left: _ -> [w340]
    shift-right: [w342] -> _
    shift-left: w5 -> [w341]
    shift-right: [w335] -> _
    shift-left: _ -> [w339]
    tunnel: w2 -> [w338]
    shift-right: [w337] -> _
    shift-left: _ -> [w336]
    stop <- w352 stop-if-true
    n168 = Preview Queue Element(queue=w347, timeout in ms (-1)=w351) -> (queue out=w353:refnum<queue>, element=w357:string)  [unwired: 1 in, 2 out]
    n169 = Match Pattern(string=w357, regular expression=":") -> (before substring=w355:string, after substring=w354:string)  [unwired: 1 in, 2 out]
    n170 = case shown="\"idle\", Default" w355 {
      tunnel: w354 -> [_ _ _ _]
      tunnel: w353 -> [_ w418 w429 w437]
      tunnel: [_ TRUE _ _] -> w352
      tunnel: [0 _ -1 0] -> w350
      tunnel: [w384 w414 w428 w438] -> w349
      tunnel: w348 -> [w382 w414 w425 w445]
      tunnel: [w385 w413 refnum<k21> refnum ("task out") w439] -> w346
      tunnel: w345 -> [w383 w413 w426 _]
      tunnel: w344 -> [w386 _ _ _]
      tunnel: [w380 w411 w421 w434] -> w343
      tunnel: [w379 w412 w422 w435] -> w342
      tunnel: w341 -> [w377 w412 w422 w435]
      tunnel: w340 -> [w378 w411 w421 w434]
      tunnel: [w376 w410 w420 w433] -> w335
      tunnel: w339 -> [w375 w410 w420 w433]
      tunnel: w338 -> [_ w407 _ _]
      tunnel: [w364 w406 w419 w431] -> w337
      tunnel: w336 -> [w363 w406 w419 w431]
      frame "idle", Default {
        n171 = Dequeue Element(queue=w386, timeout in ms (-1)=0) -> (element=w381:dbl, timed out?=w365:bool)  [unwired: 1 in, 2 out]
        n172 = case shown="True" w365 {
          tunnel: w381 -> [w396 _]
          tunnel: [w396 w398] -> w374
          tunnel: [w396 w400] -> w380
          tunnel: [w390 w405] -> w379
          tunnel: w378 -> [w395 w400]
          tunnel: w377 -> [w394 w405]
          tunnel: [w391 w402] -> w376
          tunnel: w375 -> [_ w402]
          tunnel: [w390 w397] -> w364
          frame False {
            n173 = call <vilib>:"High Resolution Relative Seconds.vi"() -> ("relative seconds"=w390:dbl)
            n174 = Subtract(x=w396, y=w395) -> (x-y=w393:dbl)
            n175 = Subtract(x=w390, y=w394) -> (x-y=w392:dbl)
            n176 = Divide(x=w393, y=w392) -> (x/y=w391:dbl)
          }
          frame True {
            n177 = call <vilib>:"High Resolution Relative Seconds.vi"() -> ("relative seconds"=w397:dbl)
            n178 = Subtract(x=w397, y=w405) -> (x-y=w404:dbl)
            n179 = Multiply(x=w404, y=w402) -> (x*y=w403:dbl)
            n180 = Add(x=w400, y=w403) -> (x+y=w401:dbl)
            n181 = Select(t=w401, s="interpolate output", f=w400) -> (s? t:f=w398:dbl)
          }
        }
        n182 = local read "p1 [mm]"() -> (w372:dbl)
        n183 = local read "p2 [mm]"() -> (w373:dbl)
        n184 = Subtract(x=w374, y=w372) -> (x-y=w371:dbl)
        n185 = Subtract(x=w373, y=w372) -> (x-y=w370:dbl)
        n186 = Subtract(x=w364, y=w363) -> (x-y=w362:dbl)
        n187 = Divide(x=w371, y=w370) -> (x/y=w369:dbl)
        n188 = Reciprocal(x=w362) -> ()  [unwired: 1 out]
        n189 = Multiply(x=w369, y=8.0) -> (x*y=w360:dbl)
        n190 = Increment(x=w360) -> (x+1=w359:dbl)
        "x*y" <- w359
        n191 = In Range and Coerce(upper limit=10.0, x=w359, lower limit=0.0) -> (coerced(x)=w361:dbl)  [unwired: 1 out]
        "output voltage" <- w361
        n192 = case shown="False" "Enable?" {
          tunnel: w361 -> [_ w389]
          frame False {
          }
          frame True {
            "Waveform Chart" <- w389
          }
        }
        n193 = call-poly <vilib>:"DAQmx Write.vi"("task/channels in"=w383, "data"=w361, "error in"=w382) -> ("task out"=w385:refnum<k21>, "error out"=w384:errorcluster)  [unwired: 10 in, 1 out]
      }
      frame "close" {
        n194 = Dequeue Element(queue=w418) -> (queue out=w417:refnum<queue>, error out=w416:errorcluster)  [unwired: 2 in, 2 out]
        n195 = Unbundle By Name(w407) -> ("dev2_data"=w408:refnum<queue>)
        n196 = Release Queue(queue=w417, error in (no error)=w416) -> ()  [unwired: 1 in, 3 out]
        n197 = Flush Queue(queue=w408) -> (queue out=w409:refnum<queue>)  [unwired: 1 in, 2 out]
        n198 = Release Queue(queue=w409) -> ()  [unwired: 2 in, 3 out]
      }
      frame "release" {
        n199 = Dequeue Element(queue=w429) -> ()  [unwired: 2 in, 4 out]
        n200 = call <vilib>:"DAQmx Stop Task.vi"("task/channels in"=w426, "error in"=w425) -> ("task out"=w424:refnum<k21>, "error out"=w423:errorcluster)  [unwired: 12 in]
        n201 = call <vilib>:"DAQmx Clear Task.vi"("task in"=w424, "error in"=w423) -> ("error out"=w428:errorcluster)  [unwired: 13 in]
      }
      frame "initialize" {
        w442 = -1 items=["Default"=-1, "RSE"=10083, "Differential"=10106, "Pseudodifferential"=12529] ("output terminal configuration")
        n202 = Dequeue Element(queue=w437) -> ()  [unwired: 2 in, 4 out]
        n203 = call-poly <vilib>:"DAQmx Create Virtual Channel.vi"("maximum value"=10.0, "minimum value"=0.0, "output terminal configuration"=w442, "physical channels"="physical channels", "error in"=w445) -> ("task out"=w441:refnum<k21>, "error out"=w440:errorcluster)  [unwired: 9 in]
        n204 = call <vilib>:"DAQmx Start Task.vi"("task/channels in"=w441, "error in"=w440) -> ("task out"=w439:refnum<k21>, "error out"=w438:errorcluster)  [unwired: 12 in]
      }
    }
    "meas. velocity" <- w335
    "DAC error" <- w349
  }
